vi "Run important tasks.vi"(6 "ControlQueue":refnum<queue>, 7 "pulses previous":dbl, 8 "error in (no error)":errorcluster, 9 "DAQmx Tasks":T1(array[cluster]), 10 "divider":i8=10, 11 "DAQmxTaskContainer in":refnum<class "DAQmxTaskContainer.lvclass">) -> (0 "error out":errorcluster, 1 "DAQmx Tasks out":T1(array[cluster]), 2 "pulses":dbl, 3 "DAQmxTaskContainer out":refnum<class "DAQmxTaskContainer.lvclass">)   [LabVIEW 2015, in "DAQmxTaskContainer.lvclass"]
uses:
  DAQmxTaskContainer.lvclass
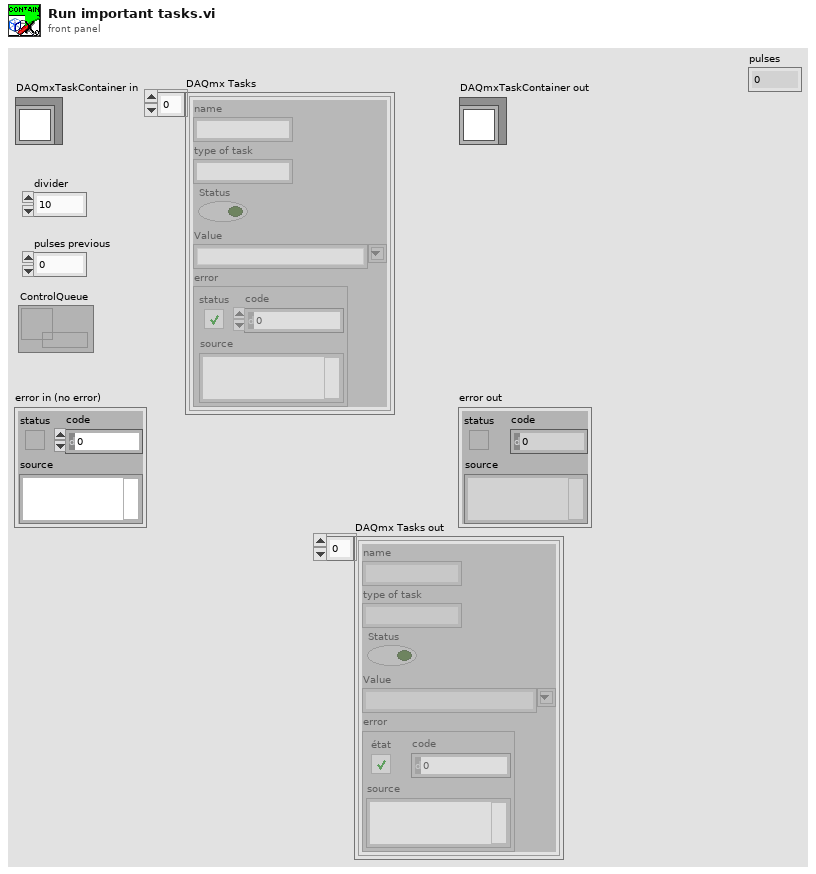
[diagram p1: front panel]
types:
  T1 = cluster{"name":string, "type of task":string, "Status":bool, "Value":string, "error":errorcluster}[]
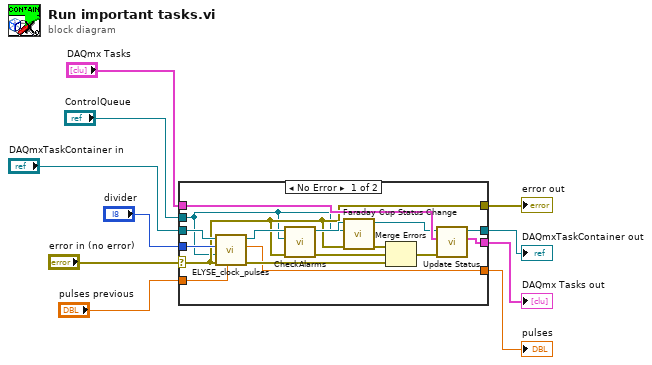
[diagram p0: block diagram]
diagram:
  n1 = case shown="No Error" "error in (no error)" {
    selector: "error in (no error)" -> [w15 w30]
    tunnel: [w15 w30] -> w9
    tunnel: [w21 w29] -> w7
    tunnel: "DAQmxTaskContainer in" -> [w22 w29]
    tunnel: "divider" -> [w20 _]
    tunnel: "ControlQueue" -> [w13 _]
    tunnel: "DAQmx Tasks" -> [w19 w28]
    tunnel: [w18 w28] -> w4
    tunnel: "pulses previous" -> [w12 w27]
    tunnel: [w11 w27] -> w1
    frame No Error {
      n2 = call "ELYSE_clock_pulses.vi"("pulses previous"=w12, "error in (no error)"=w15, "ControlQueue"=w13, "divider"=w20, "DAQmxTaskContainer en entrée"=w22) -> ("error out"=w25:errorcluster, "pulses"=w11:dbl, "DAQmxTaskContainer en sortie"=w24:refnum<class "DAQmxTaskContainer.lvclass">)  [unwired: 4 in]
      n3 = call "CheckAlarms.vi"("entrée d'erreur (pas d'erreur)"=w15, "ControlQueue"=w13, "DAQmxTaskContainer en entrée"=w24) -> ("sortie d'erreur"=w26:errorcluster, "DAQmxTaskContainer en sortie"=w17:refnum<class "DAQmxTaskContainer.lvclass">)  [unwired: 7 in]
      n4 = call "Faraday Cup Status Change.vi"("error in (no error)"=w15, "ControlQueue"=w13, "DAQmxTaskContainer in"=w17) -> ("error out"=w14:errorcluster, "DAQmxTaskContainer out"=w16:refnum<class "DAQmxTaskContainer.lvclass">)  [unwired: 7 in]
      n5 = Merge Errors(w14, w26, w25) -> (w23:errorcluster)
      n6 = call "Update Status.vi"("error in (no error)"=w23, "DAQmx Tasks"=w19, "DAQmxTaskContainer en entrée"=w16) -> ("DAQmx Tasks out"=w18:T1, "DAQmxTaskContainer en sortie"=w21:refnum<class "DAQmxTaskContainer.lvclass">)  [unwired: 6 in, 1 out]
    }
    frame Error {
    }
  }
  "error out" <- w9
  "DAQmxTaskContainer out" <- w7
  "DAQmx Tasks out" <- w4
  "pulses" <- w1
